vi "Get Name.vi"(8 "error in (no error)":errorcluster, 11 "RFFE RegWriteExtLong Command in":refnum<class "RFFE RegWriteExtLong Command.lvclass">) -> (0 "error out":errorcluster, 2 "Name":string, 3 "RFFE RegWriteExtLong Command out":refnum<class "RFFE RegWriteExtLong Command.lvclass">)   [LabVIEW 2018, in "MIPI RFFE API.lvlib" / "RFFE RegWriteExtLong Command.lvclass"]
uses:
  RFFE RegWriteExtLong Command.lvclass
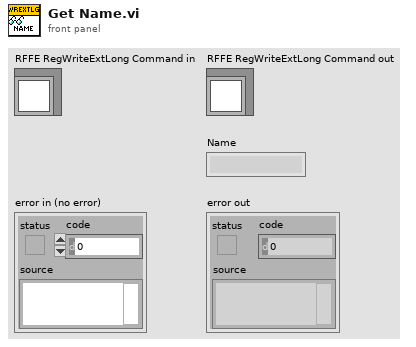
[diagram p1: front panel]
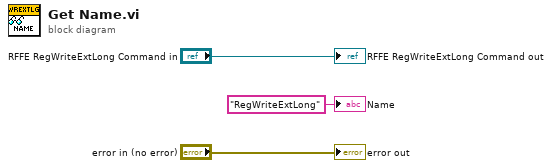
[diagram p0: block diagram]
diagram:
  "error out" <- "error in (no error)"
  "RFFE RegWriteExtLong Command out" <- "RFFE RegWriteExtLong Command in"
  "Name" <- "RegWriteExtLong" ("Name")
